vi "plot_beamCurrent_and_trip_events.vi"() -> ()   [LabVIEW 2013]
uses:
  <vilib>/addons/database/Connection.llb/DB Tools Open Connec (Path).vi
  <vilib>/addons/database/Connection.llb/Conn Execute.vi
  <vilib>/addons/database/Recordset.llb/Rec Fetch Recordset Data (R).vi
  <vilib>/addons/database/Recordset.llb/Rec Destroy - Connection.vi
  <vilib>/addons/database/_DB Variant To Data/Database Variant To Data.xnode
  <vilib>/addons/database/NI_Database_API.lvlib
panel:
  out "error out 5":errorcluster
  out "BeamCurrent History 2":cluster{timestamp[], dbl[]}(graph)
  out "result 2":string
  out "recordset data 2":variant[][](array[variant])
  out "Waveform Graph 4":dbl[](graph)
  out "Waveform Graph 3":dbl[](graph)
  out "Waveform Graph 2":dbl[](graph)
  out "Waveform Graph":dbl[](graph)
  out "recordset data":variant[][](array[variant])
  out "result":string
  out "BeamCurrent History":cluster{timestamp[], dbl[]}(graph)
  out "error out 4":errorcluster
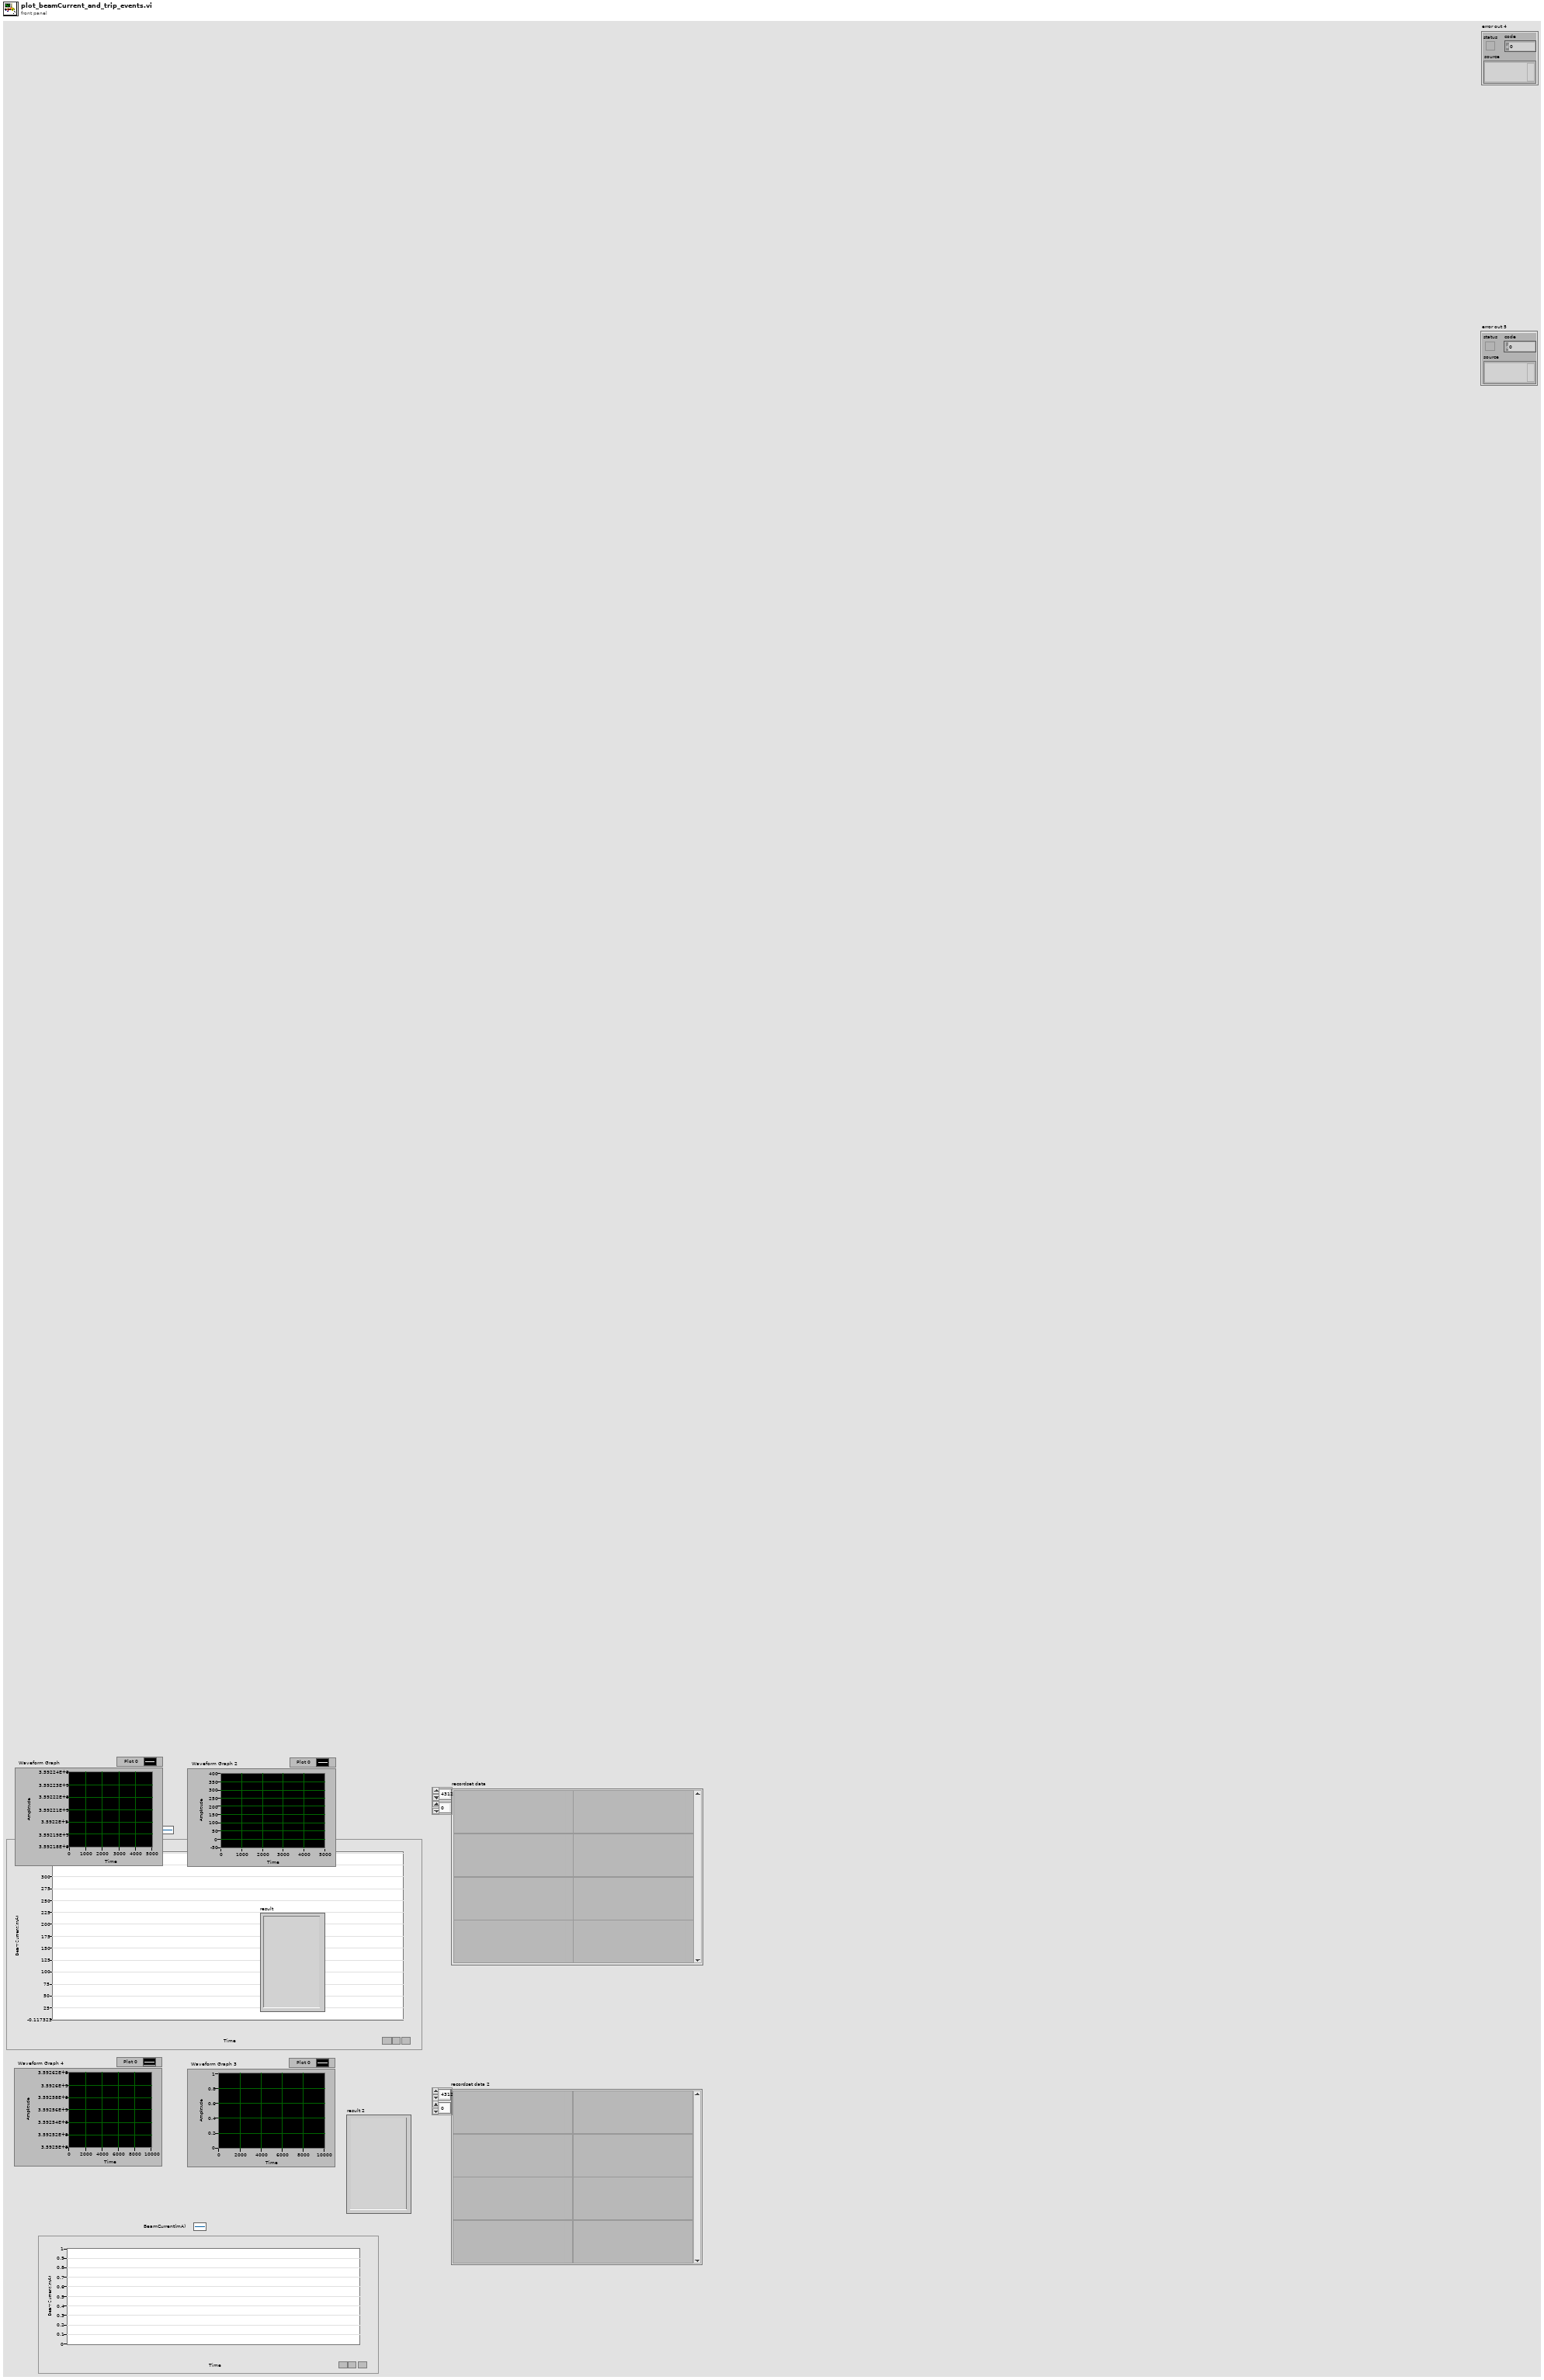
[diagram p1: front panel]
types:
  T1 = typedef "NI_Database_API.lvlib/Conn ObjectReference.ctl" = refnum<k1>
  T2 = typedef "NI_Database_API.lvlib/Rec ObjectReference.ctl" = refnum<k1>
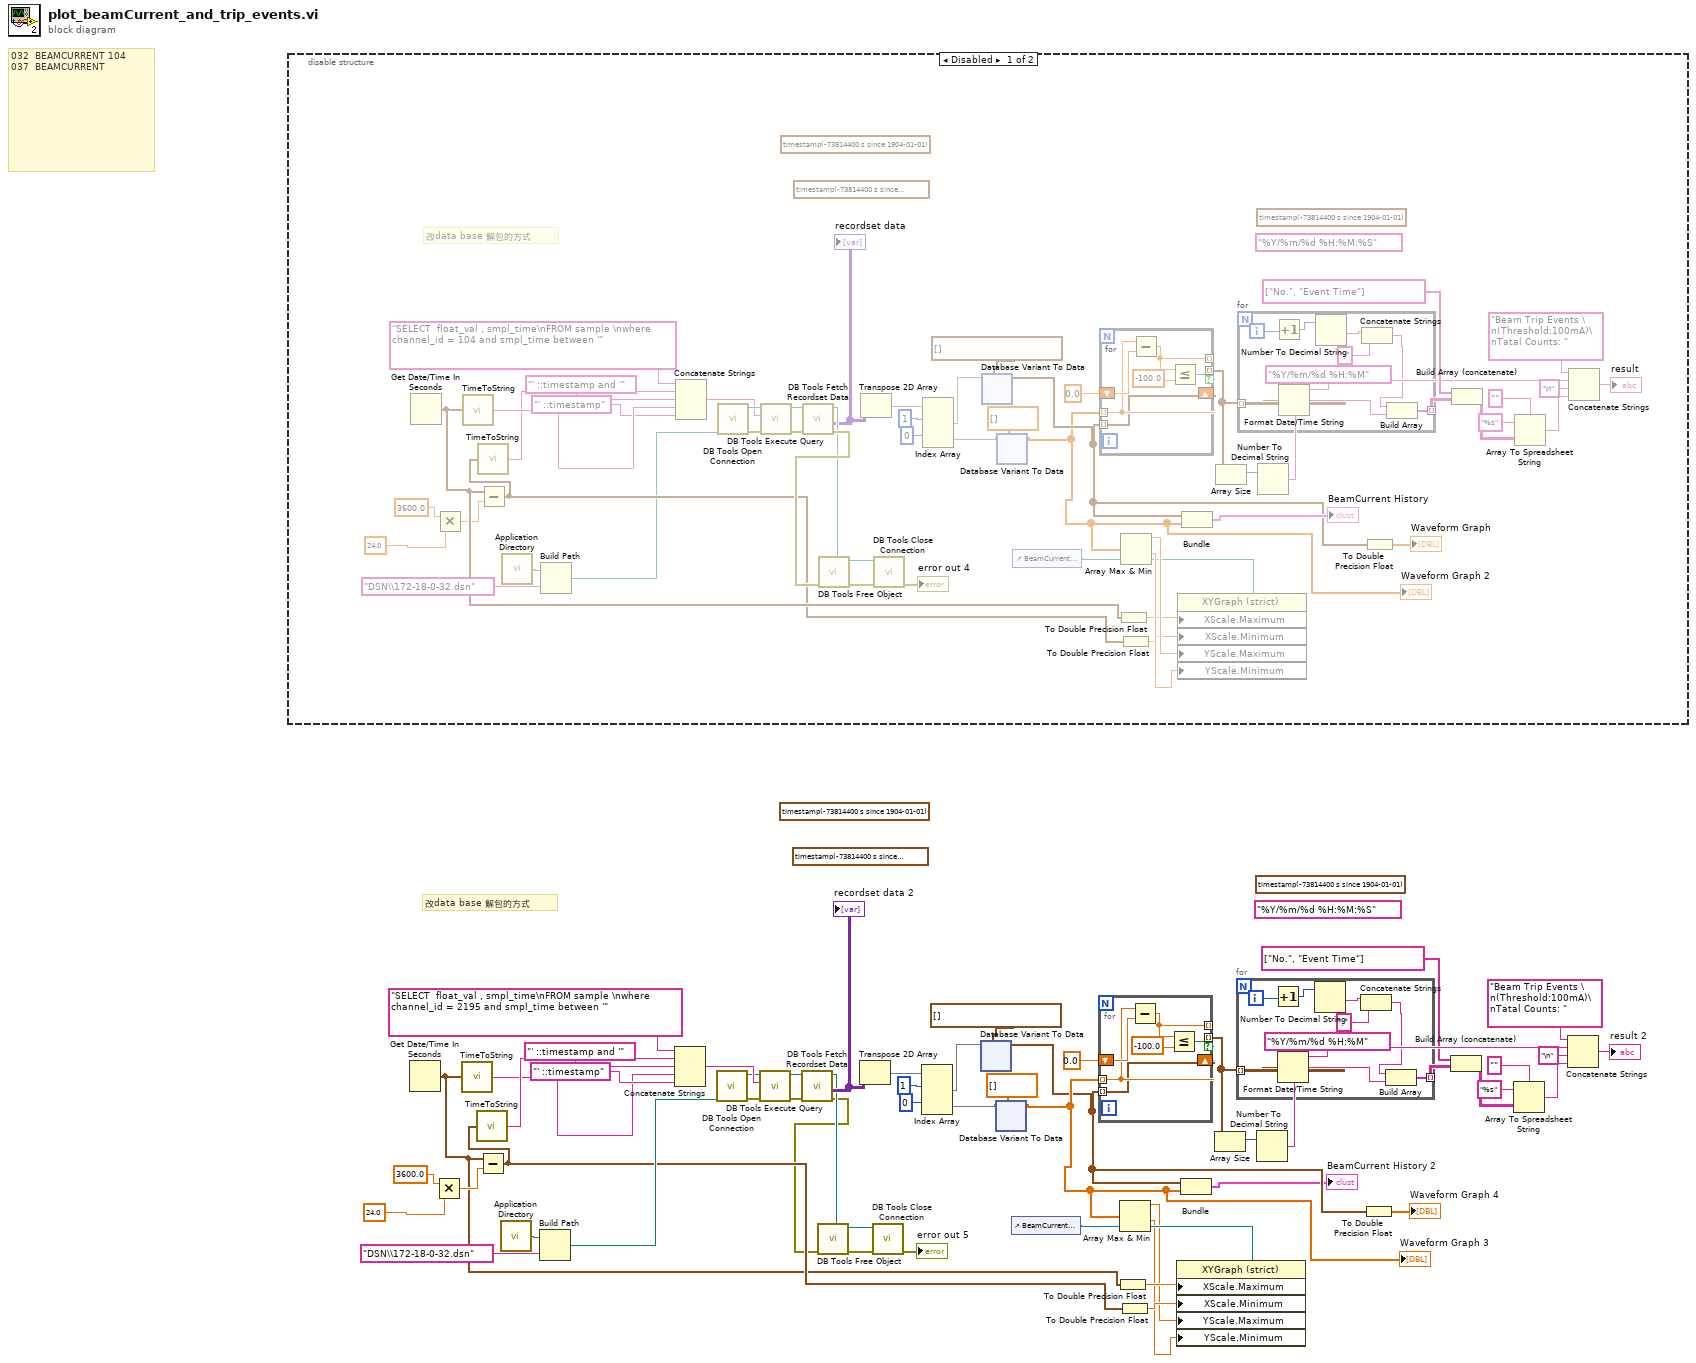
[diagram p0: block diagram]
diagram:
  (unwired) timestamp(-73814400 s since 1904-01-01)
  (unwired) timestamp(-73814400 s since 1904-01-01)
  (unwired) timestamp(-73814400 s since 1904-01-01)
  (unwired) "%Y/%m/%d %H:%M:%S" ("time format string (%c)")
  # "改data base 解包的方式"
  # "032  BEAMCURRENT 104\n037  BEAMCURRENT"
  n1 = disable-structure shown="Disabled" {
    frame Disabled {
      (unwired) timestamp(-73814400 s since 1904-01-01)
      (unwired) timestamp(-73814400 s since 1904-01-01)
      (unwired) timestamp(-73814400 s since 1904-01-01)
      (unwired) "%Y/%m/%d %H:%M:%S" ("time format string (%c)")
      # "改data base 解包的方式"
      n2 = Get Date/Time In Seconds() -> (seconds since 1Jan1904=w103:timestamp)
      n3 = Multiply(x=3600.0 ("y"), y=24.0) -> (x*y=w93:dbl)
      n4 = call "TimeToString.vi"("Time Stamp Control"=w103) -> ("result string"=w95:string)
      n5 = Subtract(x=w103, y=w93) -> (x-y=w102:timestamp)
      n6 = call "TimeToString.vi"("Time Stamp Control"=w102) -> ("result string"=w94:string)
      n7 = call <vilib>:"Application Directory.vi"() -> ("Application Directory"=w96:path)
      n8 = Build Path(base path=w96, name or relative path="DSN\\172-18-0-32.dsn") -> (appended path=w98:path)
      n9 = Concatenate Strings("SELECT  float_val , smpl_time\nFROM sample \nwhere  channel_id = 104 and smpl_time between '" ("result string"), w94, "' ::timestamp and '" ("result string"), w95, "' ::timestamp" ("result string")) -> (w81:string)
      n10 = call-poly <vilib>:"DB Tools Open Connection.vi"("connection information"=w98) -> ("error out"=w91:errorcluster, "connection reference"=w90:T1)  [unwired: 7 in]
      n11 = call-poly <vilib>:"DB Tools Execute Query.vi"("error in (no error)"=w91, "SQL query"=w81, "connection reference"=w90) -> ("error out"=w88:errorcluster, "recordset reference"=w89:T2)  [unwired: 5 in]
      n12 = call-poly <vilib>:"DB Tools Fetch Recordset Data.vi"("error in (no error)"=w88, "recordset reference"=w89) -> ("error out"=w106:errorcluster, "recordset data"=w63:variant[][], "recordset reference out"=w87:T2)  [unwired: 3 in]
      "recordset data" <- w63
      n13 = call-poly <vilib>:"DB Tools Free Object.vi"("error in (no error)"=w106, "recordset reference"=w87) -> ("error out"=w85:errorcluster, "connection reference"=w86:T1)  [unwired: 8 in]
      n14 = Transpose 2D Array(2D array=w63) -> (transposed array=w60:variant[][])
      n15 = call <vilib>:"DB Tools Close Connection.vi"("error in (no error)"=w85, "connection reference"=w86) -> ("error out"=→"error out 4":errorcluster)  [unwired: 5 in]
      n16 = Index Array(array=w60, index (row) #1=1 ("index (row)"), index (row) #2=0 ("index (row)")) -> (element #1=w58:variant[], element #2=w56:variant[])  [unwired: 2 in]
      n17 = xnode "Database Variant To Data"("database variant"=w58, "type"=timestamp[] []) -> ("data"=w57:timestamp[])  [unwired: 1 in, 1 out]
      n18 = xnode "Database Variant To Data"("database variant"=w56, "type"=dbl[] []) -> ("data"=w54:dbl[])  [unwired: 1 in, 1 out]
      "Waveform Graph 2" <- w54
      n19 = control-ref of="BeamCurrent History"() -> (w78:refnum<vi>)
      n20 = for {
        tunnel: w54 -> [w210] mode=indexing
        tunnel: w57 -> [w209] mode=indexing
        shift-right: [w210] -> _
        shift-left: 0.0 -> [w211]
        tunnel: [w209] -> w76 mode=indexing if=w208
        tunnel: [w207] -> _ mode=indexing
        n21 = Subtract(x=w210, y=w211) -> (x-y=w207:dbl)
        n22 = Less Or Equal?(x=w207, y=-100.0) -> (x <= y?=w208:bool)
      }
      n23 = To Double Precision Float(number=w103) -> (double precision float=w101:dbl)
      n24 = Array Max & Min(array=w54) -> (max value=w104:dbl, min value=w105:dbl)  [unwired: 2 out]
      n25 = To Double Precision Float(number=w102) -> (double precision float=w100:dbl)
      n26 = property on="Property Node" class="XYGraph (strict)"(reference=w78, "XScale.Maximum"=w101, "XScale.Minimum"=w100, "YScale.Maximum"=w104, "YScale.Minimum"=w105) -> ()  [unwired: 1 in, 2 out]
      n27 = Bundle("data"=w57, "data"=w54) -> (→"BeamCurrent History":cluster{"data":timestamp[], "data":dbl[]})  [unwired: 1 in]
      n28 = Array Size(array=w76) -> (size(s)=w70:i32)
      n29 = for {
        tunnel: w76 -> [w204] mode=indexing
        tunnel: [w200] -> w75 mode=indexing
        i -> [w203]
        n30 = Increment(x=w203) -> (x+1=w202:i32)
        n31 = Format Date/Time String(time format string (%c)="%Y/%m/%d %H:%M", seconds (now)=w204) -> (date/time string=w201:string)  [unwired: 1 in]
        n32 = Number To Decimal String(number=w202) -> (decimal integer string=w199:string)  [unwired: 1 in]
        n33 = Concatenate Strings(w199, "." ("string")) -> (w197:string)
        n34 = Build Array(w197, w201) -> (w200:string[])
      }
      n35 = Number To Decimal String(number=w70) -> (decimal integer string=w68:string)  [unwired: 1 in]
      n36 = To Double Precision Float(number=w57) -> (double precision float=→"Waveform Graph":dbl[])
      n37 = Build Array (concatenate)(string[] ["No.", "Event Time"], w75) -> (w71:string[][])
      n38 = Array To Spreadsheet String(delimiter (Tab)="", array=w71, 3:"%s" ("format string")) -> (spreadsheet string=w66:string)
      n39 = Concatenate Strings("Beam Trip Events \n(Threshold:100mA)\nTatal Counts: ", w68, "\n" ("string"), w66) -> (→"result":string)
    }
    frame Enabled {
    }
  }
  n40 = Get Date/Time In Seconds() -> (seconds since 1Jan1904=w4:timestamp)
  n41 = Multiply(x=3600.0 ("y"), y=24.0) -> (x*y=w14:dbl)
  n42 = call "TimeToString.vi"("Time Stamp Control"=w4) -> ("result string"=w12:string)
  n43 = Subtract(x=w4, y=w14) -> (x-y=w5:timestamp)
  n44 = call "TimeToString.vi"("Time Stamp Control"=w5) -> ("result string"=w13:string)
  n45 = call <vilib>:"Application Directory.vi"() -> ("Application Directory"=w11:path)
  n46 = Build Path(base path=w11, name or relative path="DSN\\172-18-0-32.dsn") -> (appended path=w9:path)
  n47 = Concatenate Strings("SELECT  float_val , smpl_time\nFROM sample \nwhere  channel_id = 2195 and smpl_time between '" ("result string"), w13, "' ::timestamp and '" ("result string"), w12, "' ::timestamp" ("result string")) -> (w26:string)
  n48 = call-poly <vilib>:"DB Tools Open Connection.vi"("connection information"=w9) -> ("error out"=w16:errorcluster, "connection reference"=w17:T1)  [unwired: 7 in]
  n49 = call-poly <vilib>:"DB Tools Execute Query.vi"("error in (no error)"=w16, "SQL query"=w26, "connection reference"=w17) -> ("error out"=w19:errorcluster, "recordset reference"=w18:T2)  [unwired: 5 in]
  n50 = call-poly <vilib>:"DB Tools Fetch Recordset Data.vi"("error in (no error)"=w19, "recordset reference"=w18) -> ("error out"=w1:errorcluster, "recordset data"=w44:variant[][], "recordset reference out"=w20:T2)  [unwired: 3 in]
  "recordset data 2" <- w44
  n51 = call-poly <vilib>:"DB Tools Free Object.vi"("error in (no error)"=w1, "recordset reference"=w20) -> ("error out"=w22:errorcluster, "connection reference"=w21:T1)  [unwired: 8 in]
  n52 = Transpose 2D Array(2D array=w44) -> (transposed array=w47:variant[][])
  n53 = call <vilib>:"DB Tools Close Connection.vi"("error in (no error)"=w22, "connection reference"=w21) -> ("error out"=→"error out 5":errorcluster)  [unwired: 5 in]
  n54 = Index Array(array=w47, index (row) #1=1 ("index (row)"), index (row) #2=0 ("index (row)")) -> (element #1=w49:variant[], element #2=w51:variant[])  [unwired: 2 in]
  n55 = xnode "Database Variant To Data"("database variant"=w49, "type"=timestamp[] []) -> ("data"=w50:timestamp[])  [unwired: 1 in, 1 out]
  n56 = xnode "Database Variant To Data"("database variant"=w51, "type"=dbl[] []) -> ("data"=w53:dbl[])  [unwired: 1 in, 1 out]
  "Waveform Graph 3" <- w53
  n57 = control-ref of="BeamCurrent History 2"() -> (w29:refnum<vi>)
  n58 = for {
    tunnel: w53 -> [w216] mode=indexing
    tunnel: w50 -> [w215] mode=indexing
    shift-right: [w216] -> _
    shift-left: 0.0 -> [w217]
    tunnel: [w215] -> w31 mode=indexing if=w214
    tunnel: [w213] -> _ mode=indexing
    n59 = Subtract(x=w216, y=w217) -> (x-y=w213:dbl)
    n60 = Less Or Equal?(x=w213, y=-100.0) -> (x <= y?=w214:bool)
  }
  n61 = To Double Precision Float(number=w4) -> (double precision float=w6:dbl)
  n62 = Array Max & Min(array=w53) -> (max value=w3:dbl, min value=w2:dbl)  [unwired: 2 out]
  n63 = To Double Precision Float(number=w5) -> (double precision float=w7:dbl)
  n64 = property on="Property Node" class="XYGraph (strict)"(reference=w29, "XScale.Maximum"=w6, "XScale.Minimum"=w7, "YScale.Maximum"=w3, "YScale.Minimum"=w2) -> ()  [unwired: 1 in, 2 out]
  n65 = Bundle("data"=w50, "data"=w53) -> (→"BeamCurrent History 2":cluster{"data":timestamp[], "data":dbl[]})  [unwired: 1 in]
  n66 = Array Size(array=w31) -> (size(s)=w37:i32)
  n67 = for {
    tunnel: w31 -> [w225] mode=indexing
    tunnel: [w221] -> w32 mode=indexing
    i -> [w224]
    n68 = Increment(x=w224) -> (x+1=w223:i32)
    n69 = Format Date/Time String(time format string (%c)="%Y/%m/%d %H:%M", seconds (now)=w225) -> (date/time string=w222:string)  [unwired: 1 in]
    n70 = Number To Decimal String(number=w223) -> (decimal integer string=w220:string)  [unwired: 1 in]
    n71 = Concatenate Strings(w220, "." ("string")) -> (w218:string)
    n72 = Build Array(w218, w222) -> (w221:string[])
  }
  n73 = Number To Decimal String(number=w37) -> (decimal integer string=w39:string)  [unwired: 1 in]
  n74 = To Double Precision Float(number=w50) -> (double precision float=→"Waveform Graph 4":dbl[])
  n75 = Build Array (concatenate)(string[] ["No.", "Event Time"], w32) -> (w36:string[][])
  n76 = Array To Spreadsheet String(delimiter (Tab)="", array=w36, 3:"%s" ("format string")) -> (spreadsheet string=w41:string)
  n77 = Concatenate Strings("Beam Trip Events \n(Threshold:100mA)\nTatal Counts: ", w39, "\n" ("string"), w41) -> (→"result 2":string)
